vi "N_SimuladorValores.vi"(1 "Lim Max T":dbl, 2 "Lim Min T":dbl, 3 "Numeric":i32) -> (0 "Array":dbl[](array[numeric]))   [LabVIEW 2020]
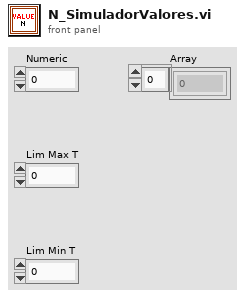
[diagram p1: front panel]
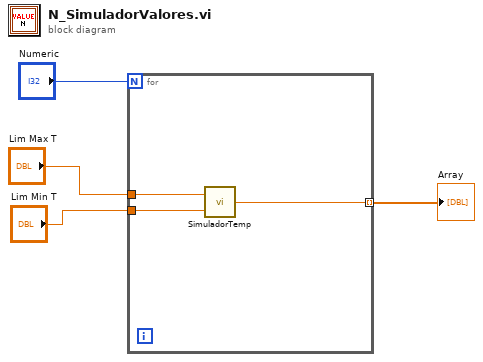
[diagram p0: block diagram]
diagram:
  n1 = for {
    N: "Numeric" -> [_]
    tunnel: "Lim Max T" -> [w7]
    tunnel: "Lim Min T" -> [w6]
    tunnel: [w5] -> w4 mode=indexing
    n2 = call "SimuladorTemp.vi"("Lim Max T"=w6, "Lim Min T"=w7) -> ("Numeric"=w5:dbl)
  }
  "Array" <- w4
